vi "Converge.vi"(0 "Maximum V_Inject":dbl format="%.4f", 1 "Tolerence":dbl format="%.2f", 2 "Power Supply Address":u8=5, 6 "Frequency Counter Address":i16=3 max=31, 7 "Minimum V_Inject":dbl format="%.4f", 9 "Nominal Frequency":dbl format="%.2f", 11 "PowerSupplyType":i32, 12 "Gate Time":T1(ring)=enum."1.0 second", 13 "Output Terminals(+6 V:0)":u16(ring) items=["+6 V output", "+25 V output", "-25 V output"], 14 "Frequency Channel":enum16{"Channel 1", "Channel 2", "Channel 3"}(ring)) -> (3 "V Limit1":dbl format="%.2f", 4 "V_Inject":dbl format="%.4f", 5 "Min Error":dbl format="%.2f", 10 "Converge OK!":bool, 15 "V Limit2":dbl format="%.2f")   [LabVIEW 2024]
panel:
  # "Input Parameters - Specified by \"c\" Runfile Command"
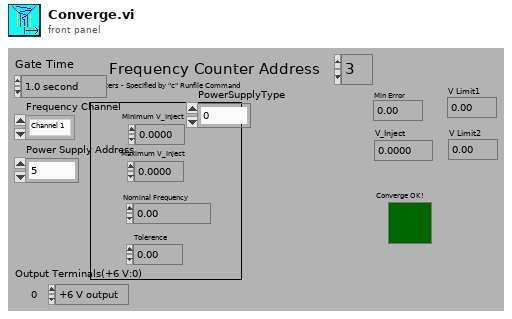
[diagram p1: front panel]
types:
  T1 = enum16{"0.1 second", "1.0 second", "10.0 second"}
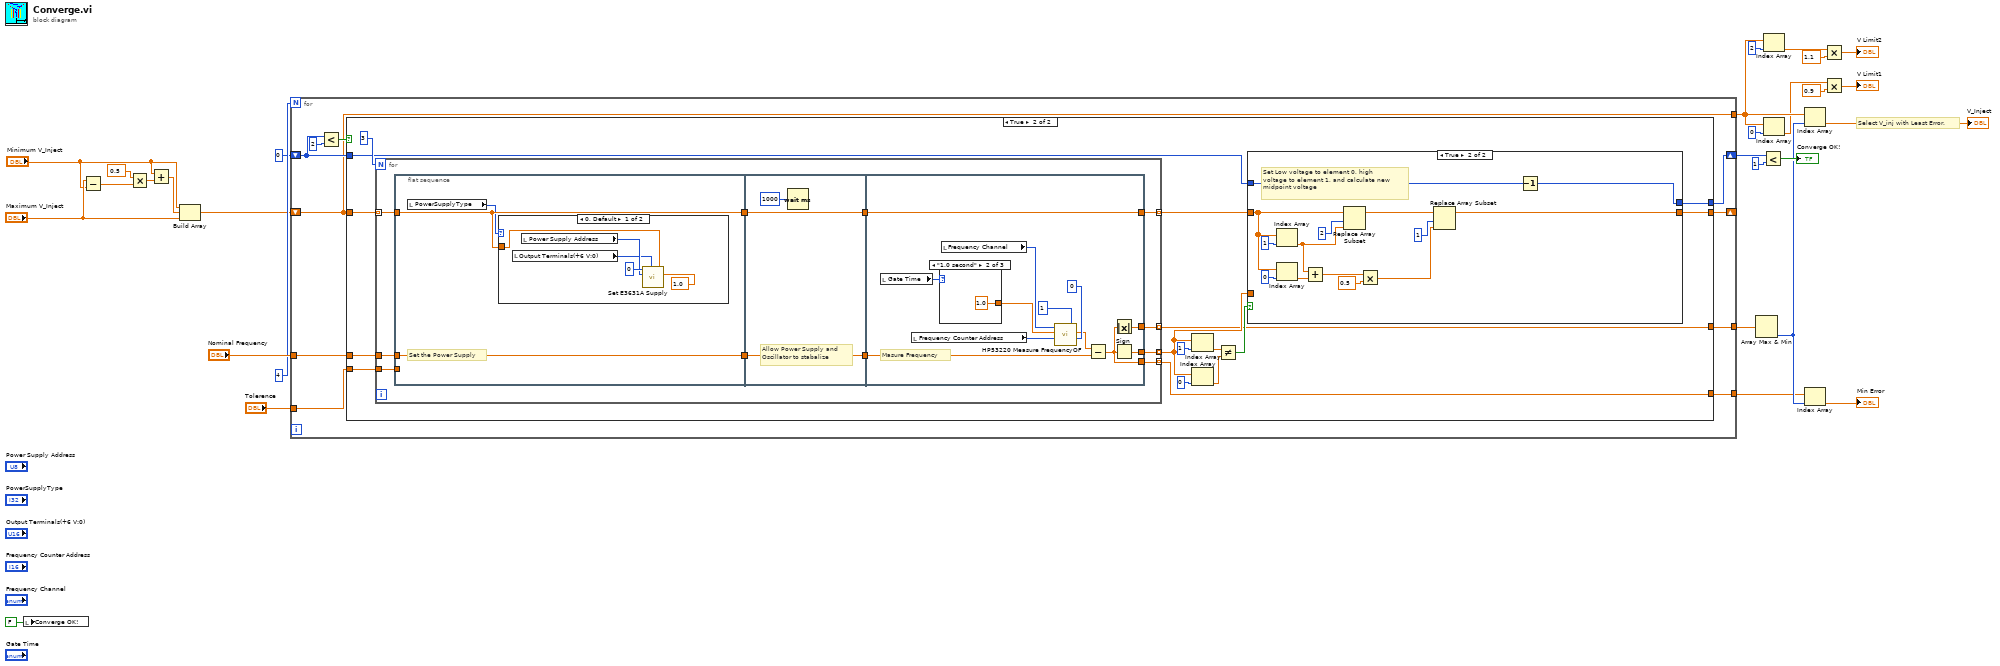
[diagram p0: block diagram]
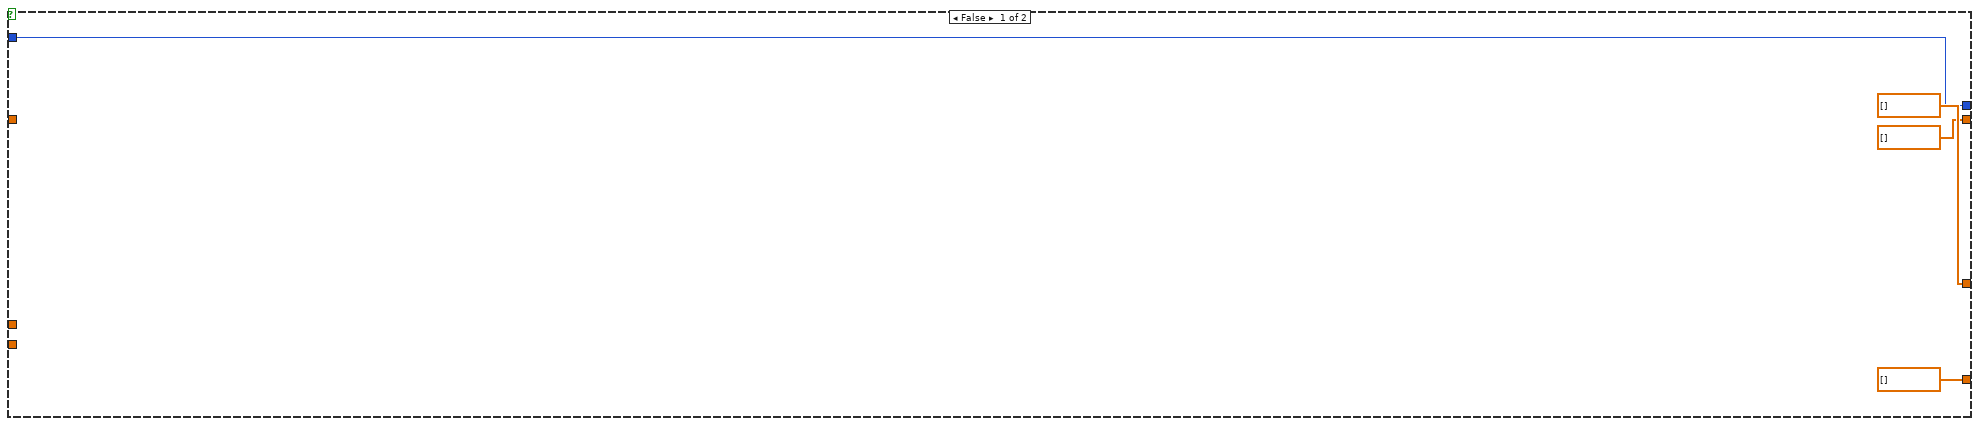
[diagram p2: hidden frame]
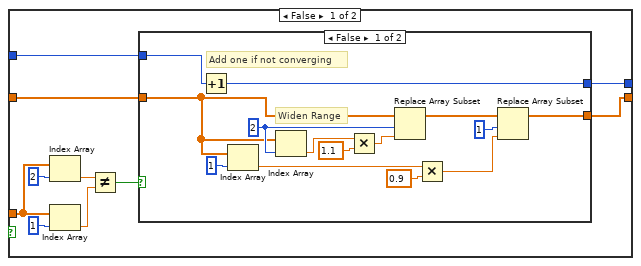
[diagram p3: hidden frame]
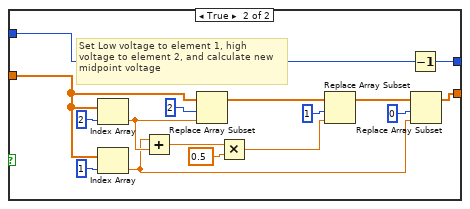
[diagram p4: hidden frame]
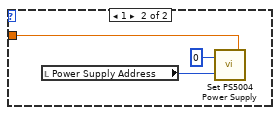
[diagram p5: hidden frame]
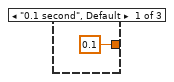
[diagram p6: hidden frame]
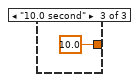
[diagram p7: hidden frame]
diagram:
  # "Select V_inj with Least Error."
  n1 = local write "Converge OK!"(FALSE ("Converge OK!")) -> ()
  n2 = Subtract(x="Maximum V_Inject", y="Minimum V_Inject") -> (x-y=w13:dbl)
  n3 = Multiply(x=0.5 ("y"), y=w13) -> (x*y=w12:dbl)
  n4 = Add(x="Minimum V_Inject", y=w12) -> (x+y=w10:dbl)
  n5 = Build Array("Minimum V_Inject", w10, "Maximum V_Inject") -> (w27:dbl[])
  n6 = for {
    N: 4 -> [_]
    tunnel: "Nominal Frequency" -> [w39]
    shift-right: [w36] -> _
    shift-left: w27 -> [w31]
    tunnel: "Tolerence" -> [w38]
    shift-right: [w37] -> w24
    shift-left: 0 -> [w32]
    tunnel: [w35] -> w21
    tunnel: [w31] -> w9
    tunnel: [w30] -> w17
    n7 = Less?(x=w32, y=i8 2) -> (x < y?=w34:bool)
    n8 = case shown="True" w34 {
      tunnel: w39 -> [_ w59]
      tunnel: w38 -> [_ w57]
      tunnel: w31 -> [_ w56]
      tunnel: w32 -> [w41 w49]
      tunnel: [w41 w48] -> w37
      tunnel: [dbl[] [] w47] -> w36
      tunnel: [dbl[] [] w44] -> w35
      tunnel: [dbl[] [] w45] -> w30
      frame False {
      }
      frame True {
        n9 = for {
          N: 3 -> [_]
          tunnel: w59 -> [w124]
          tunnel: w56 -> [w123] mode=indexing
          tunnel: w57 -> [w122]
          tunnel: [w121] -> w50 mode=indexing
          tunnel: [w120] -> w46 mode=indexing
          tunnel: [w118] -> w44 mode=indexing
          tunnel: [w119] -> w45 mode=indexing
          n10 = flat-sequence {
            tunnel: w123 -> [w126]
            tunnel: w124 -> [w127]
            tunnel: [w127] -> w117
            tunnel: w122 -> [_]
            tunnel: [w126] -> w116
            tunnel: w117 -> [w137]
            tunnel: [w137] -> w115
            tunnel: w116 -> [w136]
            tunnel: [w136] -> w114
            tunnel: [w150] -> w121
            tunnel: [w149] -> w120
            tunnel: [w148] -> w118
            tunnel: [w147] -> w119
            tunnel: w114 -> [w149]
            tunnel: w115 -> [w146]
            frame #0 {
              # "Set the Power Supply"
              n11 = local read "PowerSupplyType"() -> (w125:i32)
              n12 = case shown="0, Default" w125 {
                tunnel: w126 -> [w132 w134]
                frame 0, Default {
                  n13 = local read "Output Terminals(+6 V:0)"() -> (w129:u16)
                  n14 = local read "Power Supply Address"() -> (w130:u8)
                  n15 = call "Set E3631A Supply.vi"("Current Limit"=1.0, "Voltage Limit"=w132, "Output Terminals(+6 V:0)"=w129, "Address"=w130, "GPIB#"=u8 0) -> ()  [unwired: 3 in, 1 out]
                }
                frame 1 {
                  n16 = local read "Power Supply Address"() -> (w133:u8)
                  n17 = call "Set PS5004 Power Supply.vi"("Voltage"=w134, "Address"=w133, "System#"=0) -> ()
                }
              }
            }
            frame #1 {
              # "Allow Power Supply and \nOscillator to stabalize"
              n18 = Wait (ms)(milliseconds to wait=u32 1000) -> ()  [unwired: 1 out]
            }
            frame #2 {
              # "Masure Frequency"
              n19 = local read "Gate Time"() -> (w145:T1)
              n20 = local read "Frequency Counter Address"() -> (w143:i16)
              n21 = case shown="\"1.0 second\"" w145 {
                tunnel: [0.1 ("Gate Time") 1.0 ("Gate Time") 10.0 ("Gate Time")] -> w144
                frame "0.1 second", Default {
                }
                frame "1.0 second" {
                }
                frame "10.0 second" {
                }
              }
              n22 = local read "Frequency Channel"() -> (w140:enum16{"Channel 1", "Channel 2", "Channel 3"})
              n23 = call "HP53220 Measure FrequencyOF.vi"("GPIB Bus"=0, "Number of Readings"=1, "GPIB Address"=w143, "Gate Time"=w144, "Channel(1,2,3)"=w140) -> ("Frequency"=w139:dbl)  [unwired: 1 in, 1 out]
              n24 = Subtract(x=w139, y=w146) -> (x-y=w147:dbl)
              n25 = Absolute Value(x=w147) -> (abs(x)=w148:dbl)
              n26 = Sign(1:w147) -> (0:w150:dbl)
            }
          }
        }
        n27 = Index Array(array=w50, index=1 ("Index")) -> (element=w53:dbl)
        n28 = Index Array(array=w50, index=0 ("Index")) -> (element=w52:dbl)
        n29 = Not Equal?(x=w53, y=w52) -> (x != y?=w51:bool)
        n30 = case shown="True" w51 {
          tunnel: w46 -> [w63 w104]
          tunnel: [w62 w108] -> w47
          tunnel: w50 -> [w67 _]
          tunnel: w49 -> [w61 w106]
          tunnel: [w60 w107] -> w48
          frame False {
            n31 = Index Array(array=w67, index=2 ("Index")) -> (element=w66:dbl)
            n32 = Index Array(array=w67, index=1 ("Index")) -> (element=w65:dbl)
            n33 = Not Equal?(x=w66, y=w65) -> (x != y?=w64:bool)
            n34 = case shown="False" w64 {
              tunnel: w63 -> [w74 w90]
              tunnel: [w78 w92] -> w62
              tunnel: w61 -> [w77 w88]
              tunnel: [w76 w89] -> w60
              frame False {
                w75 = 2 ("Index")
                # "Add one if not converging"
                # "Widen Range"
                n35 = Increment(x=w77) -> (x+1=w76:i32)
                n36 = Index Array(array=w74, index=1 ("Index")) -> (element=w82:dbl)
                n37 = Index Array(array=w74, index=w75) -> (element=w71:dbl)
                n38 = Multiply(x=w71, y=1.1) -> (x*y=w70:dbl)
                n39 = Replace Array Subset(array=w74, new element=w70, index=w75) -> (w73:dbl[])
                n40 = Multiply(x=w82, y=0.9) -> (x*y=w79:dbl)
                n41 = Replace Array Subset(array=w73, new element=w79, index=1 ("Index")) -> (w78:dbl[])
              }
              frame True {
                # "Set Low voltage to element 1, high\nvoltage to element 2, and calculate new\nmidpoint voltage"
                n42 = Index Array(array=w90, index=2 ("Index")) -> (element=w87:dbl)
                n43 = Index Array(array=w90, index=1 ("Index")) -> (element=w86:dbl)
                n44 = Add(x=w86, y=w87) -> (x+y=w85:dbl)
                n45 = Replace Array Subset(array=w90, new element=w87, index=2 ("Index")) -> (w95:dbl[])
                n46 = Multiply(x=w85, y=0.5) -> (x*y=w84:dbl)
                n47 = Replace Array Subset(array=w95, new element=w84, index=1 ("Index")) -> (w93:dbl[])
                n48 = Decrement(x=w88) -> (x-1=w89:i32)
                n49 = Replace Array Subset(array=w93, new element=w86, index=0 ("Index")) -> (w92:dbl[])
              }
            }
          }
          frame True {
            # "Set Low voltage to element 0, high\nvoltage to element 1, and calculate new\nmidpoint voltage"
            n50 = Index Array(array=w104, index=1 ("Index")) -> (element=w100:dbl)
            n51 = Index Array(array=w104, index=0 ("Index")) -> (element=w101:dbl)
            n52 = Add(x=w100, y=w101) -> (x+y=w103:dbl)
            n53 = Replace Array Subset(array=w104, new element=w100, index=2 ("Index")) -> (w109:dbl[])
            n54 = Multiply(x=w103, y=0.5) -> (x*y=w102:dbl)
            n55 = Replace Array Subset(array=w109, new element=w102, index=1 ("Index")) -> (w108:dbl[])
            n56 = Decrement(x=w106) -> (x-1=w107:i32)
          }
        }
      }
    }
  }
  n57 = Array Max & Min(array=w21) -> (min index (indices)=w19:i32)  [unwired: 3 out]
  n58 = Less?(x=w24, y=1) -> (x < y?=→"Converge OK!":bool)
  n59 = Index Array(array=w9, index=2 ("Index")) -> (element=w3:dbl)
  n60 = Index Array(array=w9, index=0 ("Index")) -> (element=w6:dbl)
  n61 = Index Array(array=w9, index=w19) -> (element=→"V_Inject":dbl)
  n62 = Index Array(array=w17, index=w19) -> (element=→"Min Error":dbl)
  n63 = Multiply(x=w3, y=1.1) -> (x*y=→"V Limit2":dbl)
  n64 = Multiply(x=w6, y=0.9) -> (x*y=→"V Limit1":dbl)
